vi "Probe Generic.vi"(11 "Network Address out":refnum<class "Generic Network Address.lvclass">) -> (2 "addr":string, 3 "Boolean":bool)   [LabVIEW 2020, in "NI_WFCN.lvlib" / "Generic Network Address.lvclass"]
doc: "Prints the specific type of a Generic Network Address, and its string representation."
uses:
  <vilib>/net/WFCN/Addressing/Generic Network Address/Generic Network Address.lvclass
panel:
  out "type":string
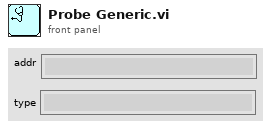
[diagram p1: front panel]
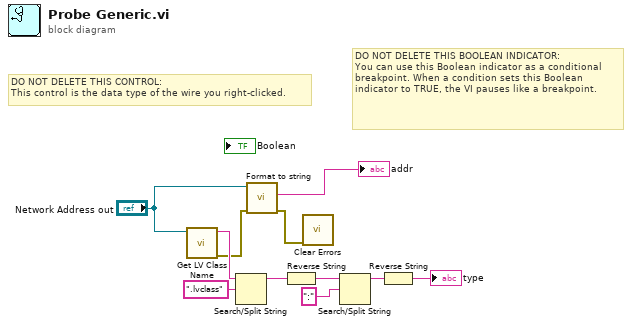
[diagram p0: block diagram]
diagram:
  # "DO NOT DELETE THIS BOOLEAN INDICATOR: \nYou can use this Boolean indicator as a conditional breakpoint. When a condition sets this Boolean indicator to TRUE, the VI pauses like a breakpoint."
  # "DO NOT DELETE THIS CONTROL: \nThis control is the data type of the wire you right-clicked."
  n1 = call <vilib>:"Get LV Class Name.vi"("object"="Network Address out") -> ("error out"=w2:errorcluster, "class name"=w9:string)  [unwired: 9 in]
  n2 = Search/Split String(string=w9, search string/char (-)=".lvclass") -> (substring before match=w7:string)  [unwired: 1 in, 2 out]
  n3 = call-dynamic "Format to string.vi"("error in (no error)"=w2, "address"="Network Address out") -> ("error out"=w1:errorcluster, "address string"=→"addr":string)  [unwired: 7 in, 1 out]
  n4 = Reverse String(1:w7) -> (0:w6:string)
  n5 = call <vilib>:"Clear Errors.vi"("error in (no error)"=w1) -> ()  [unwired: 5 in, 2 out]
  n6 = Search/Split String(string=w6, search string/char (-)=":") -> (substring before match=w4:string)  [unwired: 1 in, 2 out]
  n7 = Reverse String(1:w4) -> (0:→"type":string)
